vi "Flush Gas.vi"(7 "Display UI?":bool, 8 "error in (no error)":errorcluster, 11 "PAS":T1 caption="Gas") -> (0 "error out":errorcluster, 3 "PAS Out":T1)   [LabVIEW 2015]
uses:
  CAN Communication/PAS/Typedefs/Session Handle.ctl
  CAN Communication/PAS/PAS.lvclass
  CAN Communication/PAS/Typedefs/Valves.ctl
  User Interface/UI Handler/UI Handler.lvclass
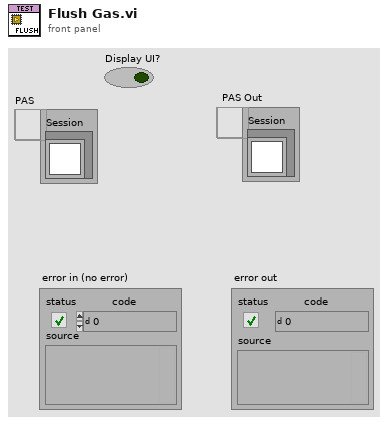
[diagram p1: front panel]
types:
  T1 = typedef "PAS.lvclass/Session Handle.ctl" = refnum<data-value>
  T2 = typedef "PAS.lvclass/Valves.ctl" = u16
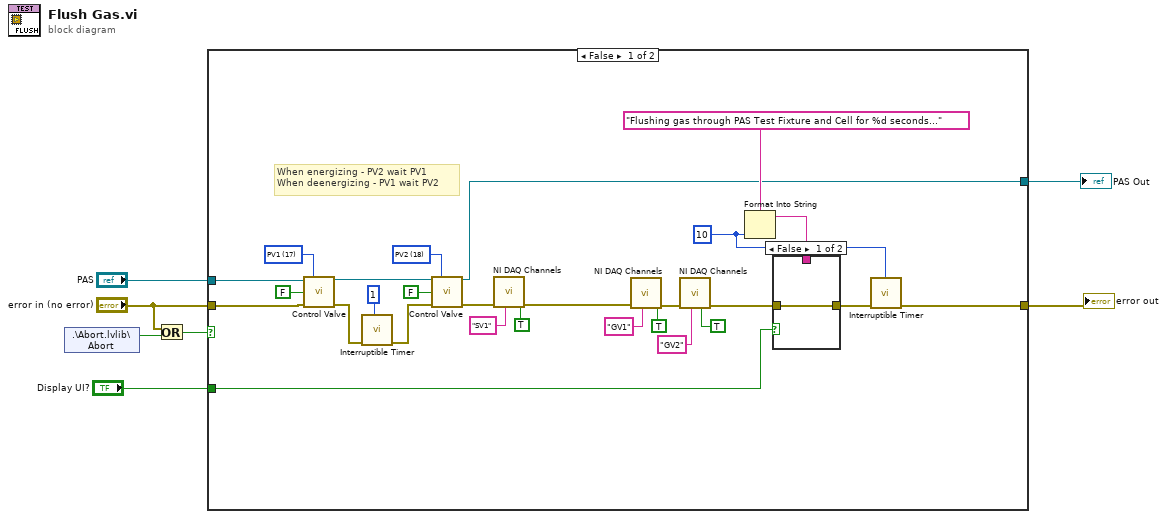
[diagram p0: block diagram]
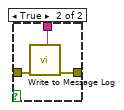
[diagram p2: hidden frame]
diagram:
  n1 = shared-variable ".\\Abort.lvlib\\Abort"() -> (w3:bool)  [unwired: 1 in, 1 out]
  n2 = Or(x="error in (no error)", y=w3) -> (x .or. y?=w2:bool)
  n3 = case shown="False" w2 {
    tunnel: [w33 w39] -> w7
    tunnel: "PAS" -> [w31 w40]
    tunnel: [w11 w40] -> w5
    tunnel: "Display UI?" -> [w10 _]
    tunnel: "error in (no error)" -> [w9 w39]
    frame False {
      w13 = 10 ("Wait (s)")
      w29 = T2 18 items=["PV1"=17, "PV2"=18, "PV3"=19, "PV4"=20] ("Valves")
      w30 = T2 17 items=["PV1"=17, "PV2"=18, "PV3"=19, "PV4"=20] ("Valves")
      # "When energizing - PV2 wait PV1\nWhen deenergizing - PV1 wait PV2"
      n4 = call "Control Valve.vi"("Session Handle in"=w31, "Valves"=w30, "Energize?"=FALSE, "error in (no error)"=w9) -> ("Session Handle out"=w27:T1, "error out"=w26:errorcluster)  [unwired: 8 in, 2 out]
      n5 = call "Interruptible Timer.vi"("error in (no error)"=w26, "Wait (s)"=1) -> ("error out"=w25:errorcluster)  [unwired: 7 in, 2 out]
      n6 = call "Control Valve.vi"("Session Handle in"=w27, "Valves"=w29, "Energize?"=FALSE, "error in (no error)"=w25) -> ("Session Handle out"=w11:T1, "error out"=w21:errorcluster)  [unwired: 8 in, 2 out]
      n7 = call "NI DAQ Channels.vi"("Control"=TRUE, "Channel"="SV1", "error in (no error)"=w21) -> ("error out"=w8:errorcluster)  [unwired: 7 in, 1 out]
      n8 = call "NI DAQ Channels.vi"("Control"=TRUE, "Channel"="GV1", "error in (no error)"=w8) -> ("error out"=w18:errorcluster)  [unwired: 7 in, 1 out]
      n9 = call "NI DAQ Channels.vi"("Control"=TRUE, "Channel"="GV2", "error in (no error)"=w18) -> ("error out"=w15:errorcluster)  [unwired: 7 in, 1 out]
      n10 = Format Into String(format string="Flushing gas through PAS Test Fixture and Cell for %d seconds...", w13) -> (resulting string=w12:string)  [unwired: 2 in, 1 out]
      n11 = case shown="False" w10 {
        tunnel: [w35 w38] -> w34
        tunnel: w15 -> [w35 w37]
        tunnel: w12 -> [_ w36]
        frame False {
        }
        frame True {
          n12 = call "Write to Message Log.vi"("error in (no error)"=w37, "Message"=w36) -> ("error out"=w38:errorcluster)  [unwired: 9 in]
        }
      }
      n13 = call "Interruptible Timer.vi"("error in (no error)"=w34, "Wait (s)"=w13) -> ("error out"=w33:errorcluster)  [unwired: 7 in, 2 out]
    }
    frame True {
    }
  }
  "error out" <- w7
  "PAS Out" <- w5
